vi "flat_loops_example.vi"() -> ()   [LabVIEW 2015]
panel:
  in  "Begin":bool
  out "Boolean":bool
  out "Numeric":dbl
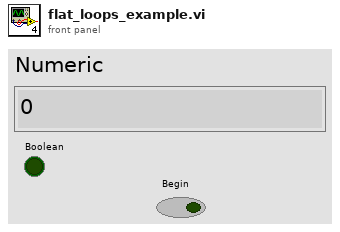
[diagram p1: front panel]
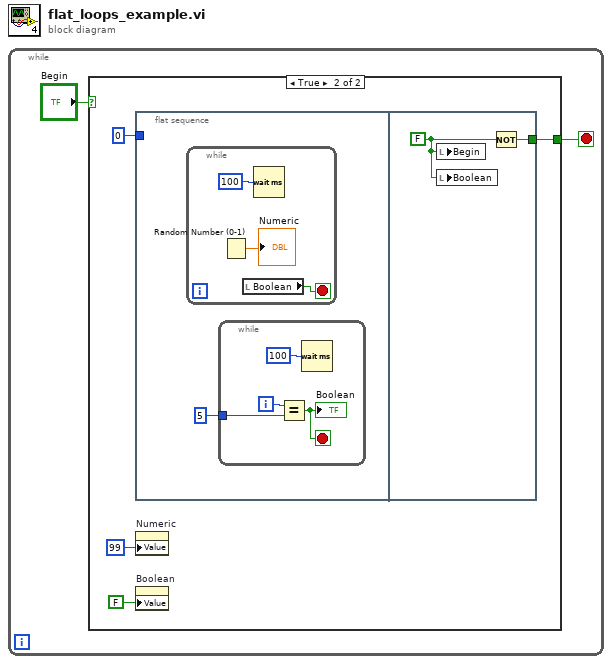
[diagram p0: block diagram]
diagram:
  n1 = while {
    stop <- w1 stop-if-true
    n2 = case shown="True" "Begin" {
      tunnel: [_ w3] -> w1
      frame False {
      }
      frame True {
        n3 = flat-sequence {
          tunnel: 0 -> [_]
          tunnel: [w15] -> w3
          frame #0 {
            n4 = while {
              stop <- w13 stop-if-true
              n5 = Random Number (0-1)() -> (number: 0 to 1=→"Numeric":dbl)
              n6 = local read "Boolean"() -> (w13:bool)
              n7 = Wait (ms)(milliseconds to wait=u32 100) -> ()  [unwired: 1 out]
            }
            n8 = while {
              tunnel: 5 -> [w9]
              i -> [w10]
              stop <- w8 stop-if-true
              n9 = Equal?(x=w10, y=w9) -> (x = y?=w8:bool)
              "Boolean" <- w8
              n10 = Wait (ms)(milliseconds to wait=u32 100) -> ()  [unwired: 1 out]
            }
          }
          frame #1 {
            w16 = FALSE
            n11 = local write "Begin"(w16) -> ()
            n12 = local write "Boolean"(w16) -> ()
            n13 = Not(x=w16) -> (.not. x?=w15:bool)
          }
        }
        n14 = property on="Numeric" class="DigNum (strict)"("Value"=99) -> ()  [unwired: 2 in, 2 out]
        n15 = property on="Boolean" class="Bool (strict)"("Value"=FALSE) -> ()  [unwired: 2 in, 2 out]
      }
    }
  }
